vi "PositionControl.vi"(4 "deadband":dbl, 5 "maxdemand":dbl, 6 "threshold":dbl, 7 "mindemand":dbl, 8 "Sequential Checks":dbl, 11 "Error":dbl) -> (1 "on target":bool, 3 "output variable":dbl)   [LabVIEW 2020]
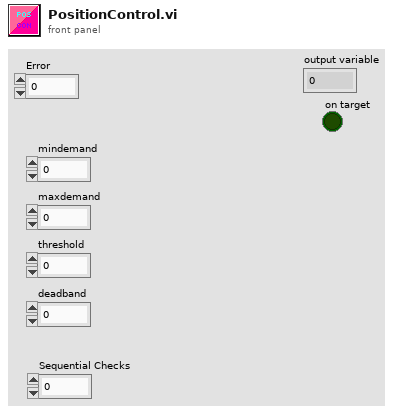
[diagram p1: front panel]
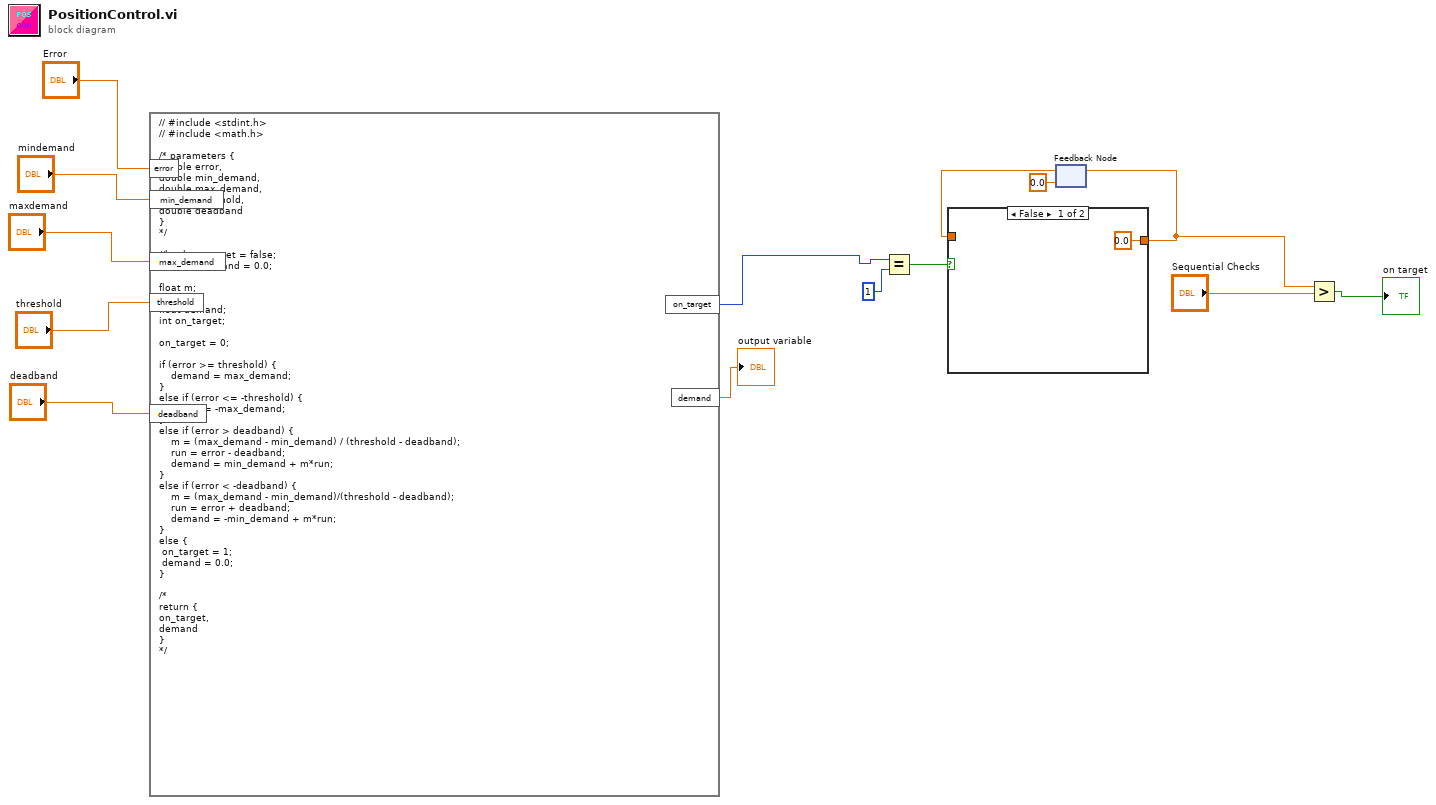
[diagram p0: block diagram]
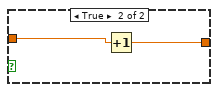
[diagram p2: hidden frame]
diagram:
  n1 = formula code="// #include <stdint.h>\n// #include <math.h>\n\n/* parameters {\ndouble error, \ndouble min_demand, \ndouble max_demand, \ndouble threshold, \ndouble deadband\n}\n*/\n\n//bool on_target = false;\n//double demand = 0.0;\n \nfloat m;\nfloat run;\nfloat demand;\nint on_target;\n\non_target = 0;\n\nif (error >= threshold) {\n   \tdemand = max_demand;\n} \nelse if (error <= -threshold) {\n\tdemand = -max_demand;\n}\nelse if (error > deadband) {\n\t   m = (max_demand - min_demand) / (threshold - deadband);\n\t   run = error - deadband;\n\t   demand = min_demand + m*run;\n}\nelse if (error < -deadband) {\n\t   m = (max_demand - min_demand)/(threshold - deadband);\n\t   run = error + deadband;\n\t   demand = -min_demand + m*run;\n}\nelse {\n\ton_target = 1;\n\tdemand = 0.0;\n}\n\n/*\nreturn {\non_target,\ndemand\n}\n*/"("error"="Error", "min_demand"="mindemand", "max_demand"="maxdemand", "threshold"="threshold", "deadband"="deadband") -> ("on_target"=w8:i32, "demand"=→"output variable":dbl)
  n2 = Equal?(x=w8, y=1) -> (x = y?=w6:bool)
  n3 = feedback #1(0.0) -> (w5:dbl)
  n4 = case shown="False" w6 {
    tunnel: w5 -> [_ w17]
    tunnel: [0.0 w16] -> w3
    frame False {
    }
    frame True {
      n5 = Increment(x=w17) -> (x+1=w16:dbl)
    }
  }
  n6 = feedback-in #1(w3) -> ()
  n7 = Greater?(x=w3, y="Sequential Checks") -> (0:→"on target":bool)
